vi "Find Target Item.vi"(7 "Type":string, 8 "error in (no error)":errorcluster, 10 "Target Item Name":string, 11 "TargetItem in":refnum<vi>) -> (0 "error out":errorcluster, 1 "Found ?":bool, 2 "Item out":refnum<vi>, 3 "TargetItem out":refnum<vi>)   [LabVIEW 2019, in "Project Sync Tools.lvclass"]
uses:
  Project Sync Tools.lvclass
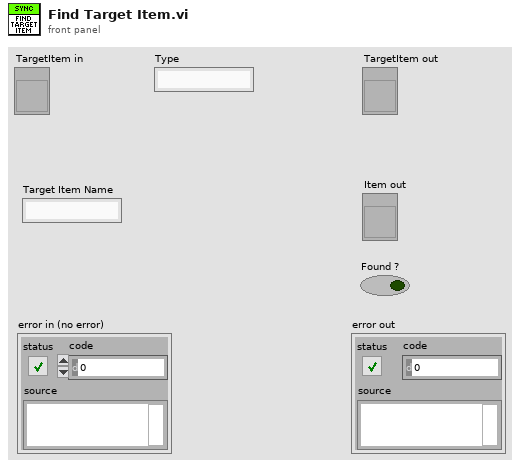
[diagram p1: front panel]
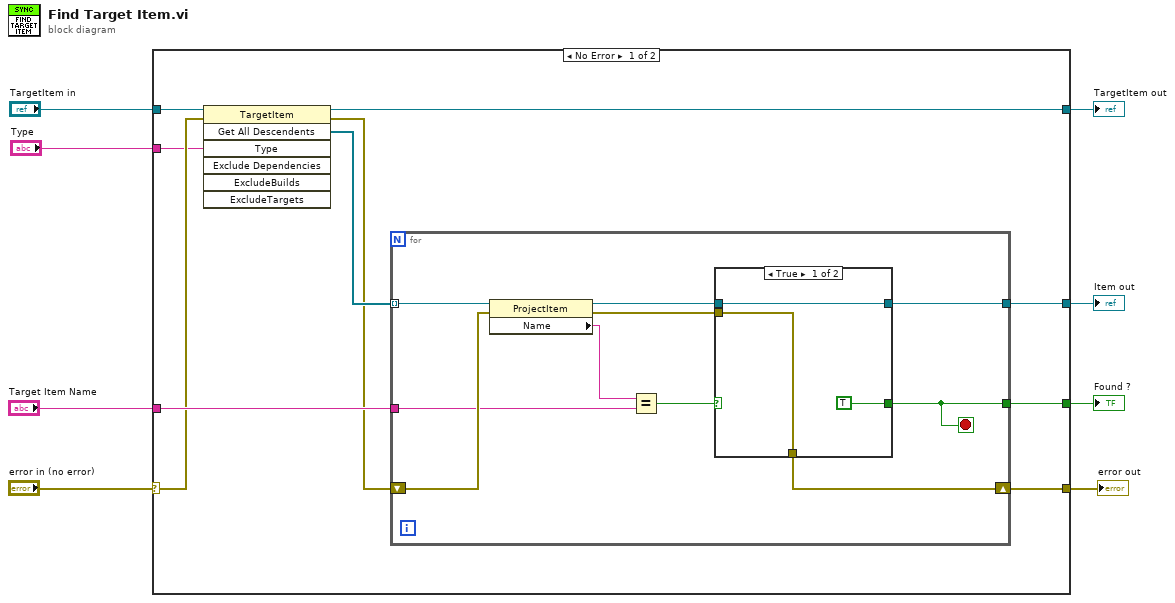
[diagram p0: block diagram]
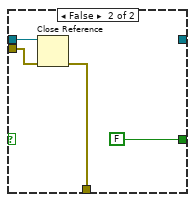
[diagram p2: hidden frame]
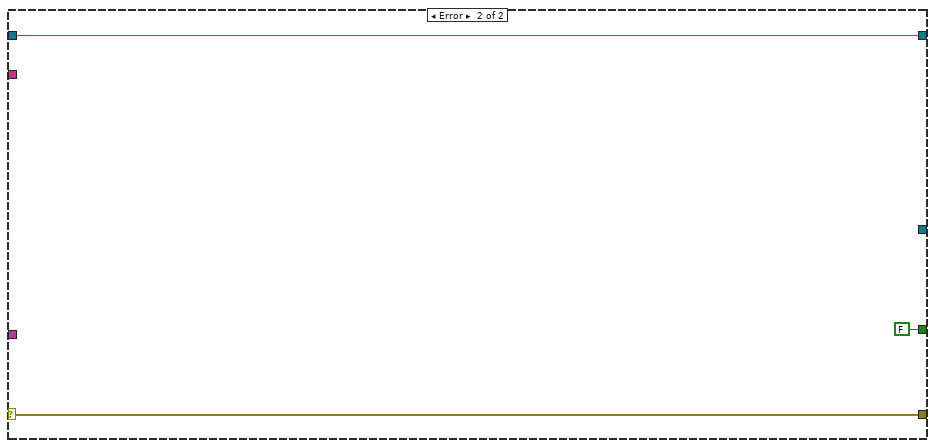
[diagram p3: hidden frame]
diagram:
  n1 = case shown="No Error" "error in (no error)" {
    selector: "error in (no error)" -> [w12 w36]
    tunnel: [w18 _] -> w8
    tunnel: [w17 FALSE] -> w7
    tunnel: "Target Item Name" -> [w16 _]
    tunnel: [w15 w36] -> w5
    tunnel: "TargetItem in" -> [w14 w38]
    tunnel: [w13 w38] -> w3
    tunnel: "Type" -> [w9 _]
    frame No Error {
      n2 = invoke class="TargetItem" method="Get All Descendents"(reference=w14, error in=w12, "Type"=w9) -> (reference out=w13:refnum<vi>, error out=w10:errorcluster, "All Descendents"=w11:refnum<vi>[])  [unwired: 4 in, 4 out]
      n3 = for {
        tunnel: w11 -> [w23] mode=indexing
        shift-right: [w25] -> w15
        shift-left: w10 -> [w28]
        tunnel: [w24] -> w17
        tunnel: [w22] -> w18
        tunnel: w16 -> [w21]
        stop <- w24 stop-if-true
        n4 = property class="ProjectItem"(reference=w23, error in=w28) -> (reference out=w27:refnum<vi>, error out=w26:errorcluster, "Name"=w20:string)
        n5 = Equal?(x=w20, y=w21) -> (x = y?=w19:bool)
        n6 = case shown="True" w19 {
          tunnel: w27 -> [w29 w35]
          tunnel: w26 -> [w31 w34]
          tunnel: [w31 w32] -> w25
          tunnel: [TRUE FALSE] -> w24
          tunnel: [w29 _] -> w22
          frame True {
          }
          frame False {
            n7 = Close Reference(reference=w35, error in (no error)=w34) -> (error out=w32:errorcluster)
          }
        }
      }
    }
    frame Error {
    }
  }
  "Item out" <- w8
  "Found ?" <- w7
  "error out" <- w5
  "TargetItem out" <- w3
